vi "Report Init.vi"(8 "error in (no error)":errorcluster, 11 "report":T1) -> (0 "error out":errorcluster, 3 "report out":T1)   [LabVIEW 2017, in "WebServiceImporter.lvlib" / "Error Handling.lvlib"]
uses:
  <vilib>/Platform/WebService/Error Handling/Error Handling.lvlib
  <resource>/importtools/NISH Report/Generate Report Object Reference.ctl
  <vilib>/Platform/WebService/Global/Const Strings.vi
  <resource>/importtools/NISH Report/NISH Report.lvlib
  <vilib>/Platform/WebService/ProxyDll Generator/ProxyDll Generator.lvlib
  <vilib>/Platform/WebService/WebServiceImporter.lvlib
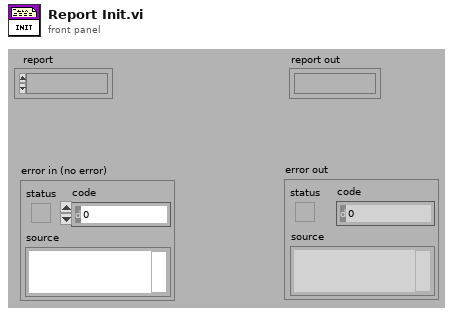
[diagram p1: front panel]
types:
  T1 = typedef "NISH Report.lvlib/Generate Report Object Reference.ctl" = refnum<k1>
  T2 = cluster{"Charset (-1)":i16, "Weight (-1)":i16, "Name":string, "Size":string}
  T3 = cluster{"Italic":enum16{"Italic Unchanged", "Italic On", "Italic Off"}, "Strike Through":enum16{"Strike Through Unchanged", "Strike Through On", "Strike Through Off"}, "Underline":enum16{"Underline Unchanged", "Underline On", "Underline Off"}, "Bold":enum16{"Bold Unchanged", "Bold On", "Bold Off"}}
  T4 = cluster{"top":dbl, "left":dbl, "right":dbl, "bottom":dbl}
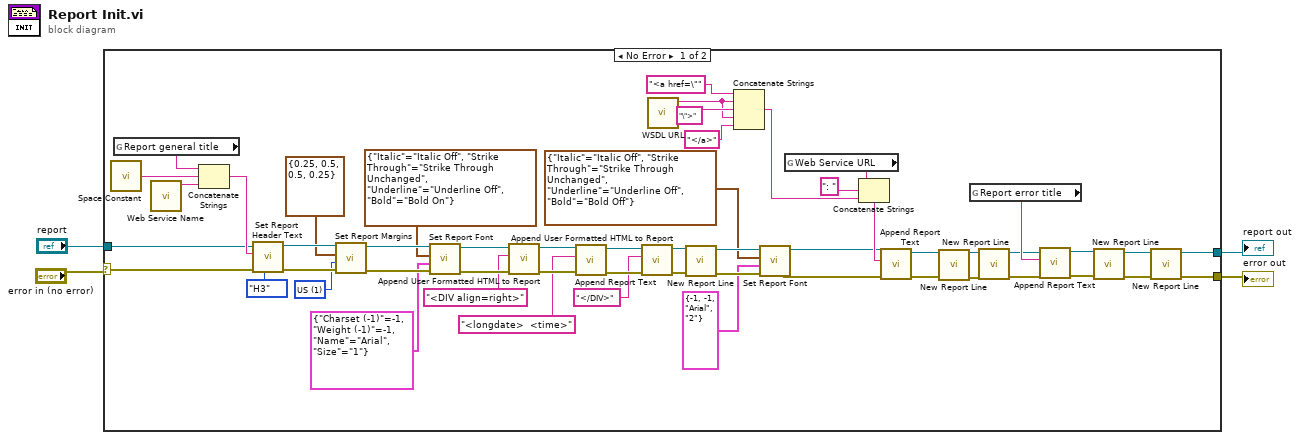
[diagram p0: block diagram]
diagram:
  n1 = case shown="No Error" "error in (no error)" {
    selector: "error in (no error)" -> [w54 w59]
    tunnel: "report" -> [w55 w58]
    tunnel: [w26 w59] -> w2
    tunnel: [w25 w58] -> w1
    frame No Error {
      w52 = u16 1 items=["Default", "US", "Metric"] ("measurement system (Default)")
      n2 = call <vilib>:"Space Constant.vi"() -> ("String"=w5:string)
      n3 = global read "Const Strings.vi" "Report general title"() -> (w24:string)
      n4 = call <vilib>:"Web Service Name.vi"() -> ("Web Service Name (out)"=w6:string)  [unwired: 10 in, 1 out]
      n5 = Concatenate Strings(w24, w5, w6) -> (w56:string)
      n6 = call <resource>:"Set Report Header Text.vi"("HTML header size"=enum16{"H1", "H2", "H3", "H4", "H5", "H6", "H7"}."H3", "error in (no error)"=w54, "center header text"=w56, "report in"=w55) -> ("error out"=w53:errorcluster, "report out"=w51:T1)  [unwired: 6 in]
      n7 = call <resource>:"Set Report Margins.vi"("error in (no error)"=w53, "measurement system (Default)"=w52, "margins (1.00)"=T4 {"top"=0.25, "left"=0.5, "right"=0.5, "bottom"=0.25}, "report in"=w51) -> ("error out"=w49:errorcluster, "report out"=w48:T1)  [unwired: 2 in]
      n8 = call <resource>:"Set Report Font.vi"("error in (no error)"=w49, "font settings"=T2 {"Charset (-1)"=-1, "Weight (-1)"=-1, "Name"="Arial", "Size"="1"} ("Font Settings"), "text options"=T3 {"Italic"=enum."Italic Off", "Strike Through"=enum."Strike Through Unchanged", "Underline"=enum."Underline Off", "Bold"=enum."Bold On"} ("Text Options"), "report in"=w48) -> ("error out"=w44:errorcluster, "report out"=w45:T1)  [unwired: 3 in]
      n9 = call <resource>:"Append User Formatted HTML to Report.vi"("error in (no error)"=w44, "HTML text"="<DIV align=right>" ("right header text"), "report in"=w45) -> ("error out"=w41:errorcluster, "report out"=w42:T1)  [unwired: 3 in]
      n10 = call <resource>:"Append Report Text.vi"("error in (no error)"=w41, "text"="<longdate>  <time>", "report in"=w42) -> ("error out"=w39:errorcluster, "report out"=w38:T1)  [unwired: 3 in]
      n11 = call <resource>:"Append User Formatted HTML to Report.vi"("error in (no error)"=w39, "HTML text"="</DIV>", "report in"=w38) -> ("error out"=w35:errorcluster, "report out"=w36:T1)  [unwired: 3 in]
      n12 = call <vilib>:"WSDL URL.vi"() -> ("WSDL URL (out)"=w9:string)  [unwired: 10 in, 1 out]
      n13 = call <resource>:"New Report Line.vi"("error in (no error)"=w35, "report in"=w36) -> ("error out"=w34:errorcluster, "report out"=w33:T1)  [unwired: 4 in]
      n14 = Concatenate Strings("<a href=\"", w9, "\">", w9, "</a>" ("string")) -> (w7:string)
      n15 = call <resource>:"Set Report Font.vi"("error in (no error)"=w34, "font settings"=T2 {"Charset (-1)"=-1, "Weight (-1)"=-1, "Name"="Arial", "Size"="2"} ("Font Settings"), "text options"=T3 {"Italic"=enum."Italic Off", "Strike Through"=enum."Strike Through Unchanged", "Underline"=enum."Underline Off", "Bold"=enum."Bold Off"} ("Text Options"), "report in"=w33) -> ("error out"=w17:errorcluster, "report out"=w12:T1)  [unwired: 3 in]
      n16 = global read "Const Strings.vi" "Web Service URL"() -> (w14:string)
      n17 = Concatenate Strings(w14, ": " ("string"), w7) -> (w15:string)
      n18 = call <resource>:"Append Report Text.vi"("error in (no error)"=w17, "text"=w15, "report in"=w12) -> ("error out"=w18:errorcluster, "report out"=w16:T1)  [unwired: 3 in]
      n19 = call <resource>:"New Report Line.vi"("error in (no error)"=w18, "report in"=w16) -> ("error out"=w21:errorcluster, "report out"=w19:T1)  [unwired: 4 in]
      n20 = global read "Const Strings.vi" "Report error title"() -> (w23:string)
      n21 = call <resource>:"New Report Line.vi"("error in (no error)"=w21, "report in"=w19) -> ("error out"=w22:errorcluster, "report out"=w20:T1)  [unwired: 4 in]
      n22 = call <resource>:"Append Report Text.vi"("error in (no error)"=w22, "text"=w23, "report in"=w20) -> ("error out"=w28:errorcluster, "report out"=w27:T1)  [unwired: 3 in]
      n23 = call <resource>:"New Report Line.vi"("error in (no error)"=w28, "report in"=w27) -> ("error out"=w30:errorcluster, "report out"=w29:T1)  [unwired: 4 in]
      n24 = call <resource>:"New Report Line.vi"("error in (no error)"=w30, "report in"=w29) -> ("error out"=w26:errorcluster, "report out"=w25:T1)  [unwired: 4 in]
    }
    frame Error {
    }
  }
  "error out" <- w2
  "report out" <- w1
